vi "Dynamic Load Labjack.vi"(8 "error in":errorcluster) -> (0 "error out":errorcluster, 3 "Instrument Driver":refnum<class "Instrument Driver.lvclass">)   [LabVIEW 2021]
uses:
  Instrument Driver/Instrument Driver.lvclass
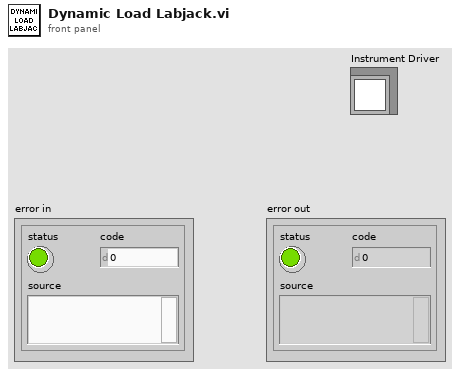
[diagram p1: front panel]
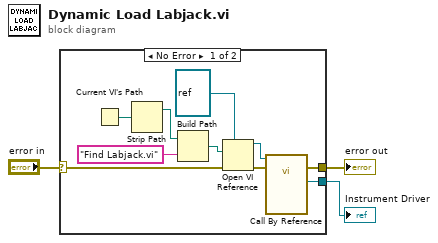
[diagram p0: block diagram]
diagram:
  n1 = case shown="No Error" "error in" {
    selector: "error in" -> [w9 w14]
    tunnel: [w5 _] -> w2
    tunnel: [w4 w14] -> w1
    frame No Error {
      n2 = Current VI's Path() -> (path=w13:path)
      n3 = Strip Path(path=w13) -> (stripped path=w12:path)  [unwired: 1 out]
      n4 = Build Path(base path=w12, name or relative path="Find Labjack.vi") -> (appended path=w10:path)
      n5 = Open VI Reference(type specifier VI Refnum (for type only)=refnum<vi> refnum, vi path=w10, error in (no error)=w9) -> (vi reference=w6:refnum<vi>, error out=w7:errorcluster)  [unwired: 3 in]
      n6 = call-by-ref "?"(reference=w6, error in=w7) -> (error out=w4:errorcluster, "Instrument Driver"=w5:refnum<class "Instrument Driver.lvclass">)  [unwired: 11 in, 1 out]
    }
    frame Error {
    }
  }
  "error out" <- w1
  "Instrument Driver" <- w2
